vi "Frame_CRC_check.vi"(8 "error in (no error)":errorcluster, 11 "ISO 14443 A UP in":refnum<class "ISO 14443 A UP.lvclass">) -> (0 "error out":errorcluster, 3 "ISO 14443 A UP out":refnum<class "ISO 14443 A UP.lvclass">)   [LabVIEW 2019, in "ISO 14443 A UP.lvclass"]
uses:
  ISO 14443 A UP.lvclass
  ISO 14443 A UP.lvclass/ISO 14443 A UP.ctl
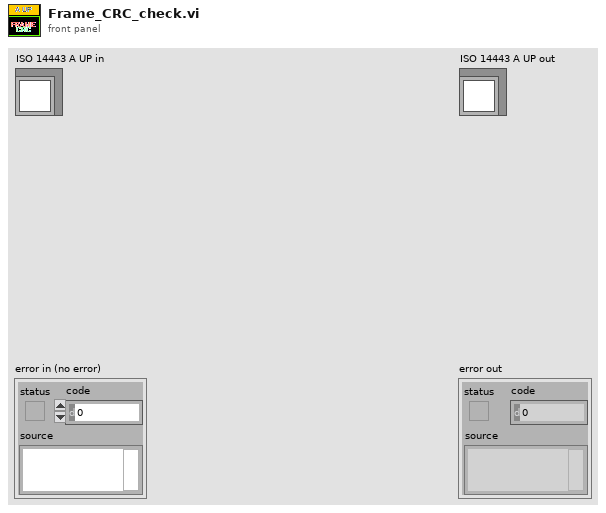
[diagram p1: front panel]
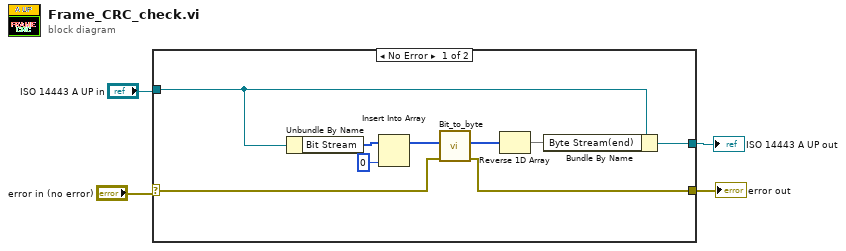
[diagram p0: block diagram]
diagram:
  n1 = case shown="No Error" "error in (no error)" {
    selector: "error in (no error)" -> [w7 w14]
    tunnel: [w6 w14] -> w2
    tunnel: "ISO 14443 A UP in" -> [w10 w15]
    tunnel: [w9 w15] -> w3
    frame No Error {
      n2 = Unbundle By Name(w10) -> ("Bit Stream"=w11:u8[])
      n3 = Insert Into Array(array=w11, new element=u8 0 ("new element/subarray")) -> (w12:u8[])  [unwired: 1 in]
      n4 = call "Bit_to_byte.vi"("Error In"=w7, "Array of bit"=w12) -> ("Error Out"=w6:errorcluster, "Array of byte"=w8:u8[])  [unwired: 7 in, 1 out]
      n5 = Reverse 1D Array(array=w8) -> (reversed array=w5:u8[])
      n6 = Bundle By Name(cluster=w10, "Byte Stream(end)"=w5) -> (w9:refnum<class "ISO 14443 A UP.lvclass">)
    }
    frame Error {
    }
  }
  "error out" <- w2
  "ISO 14443 A UP out" <- w3
